vi "Main.vi"(8 "error in":errorcluster caption="entrée d'erreur") -> (0 "error out":errorcluster caption="sortie d'erreur")   [LabVIEW 2026]
uses:
  FGV_Controls/State.ctl
  FGV_Controls/TypeDef_FGV.ctl
panel:
  in  "Delete Positions":bool
  out "Multipositions":dbl[][](array[numeric])
  in  "Add":bool
  in  "Relative movement (mm)":dbl[](array[numeric]) format="%.6f"
  in  "Set Vel":bool
  in  "Velocity values":dbl[](array[numeric]) format="%.6f"
  out "Velocity":dbl[](array[numeric]) format="%.6f"
  in  "Mode":bool
  in  "Mov Rel":bool
  in  "Mov Abs":bool
  in  "Go to (mm)":dbl[](array[numeric]) format="%.6f"
  out "Current positions":dbl[](array[numeric])
  in  "Servo mode":bool[](array[boolean])
  out "+/- movement\nrange":dbl[](array[numeric]) format="%.6f"
  in  "Stop":bool
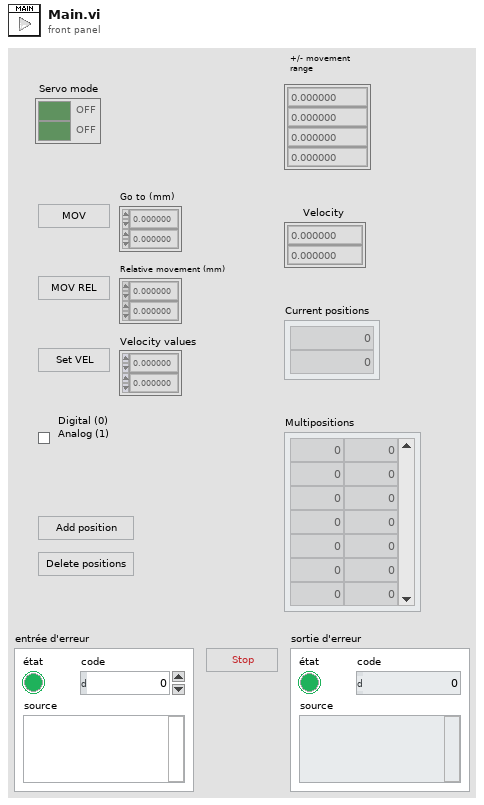
[diagram p1: front panel]
types:
  T1 = typedef "TypeDef_FGV.ctl" = enum16{"Initialize", "Write", "Read"}
  T2 = typedef "State.ctl" = enum16{"Initialize", "Wait for Event", "MOVAbs", "MOVRel", "SVO", "Analog-Digital", "POS?", "VEL", "STOP"}
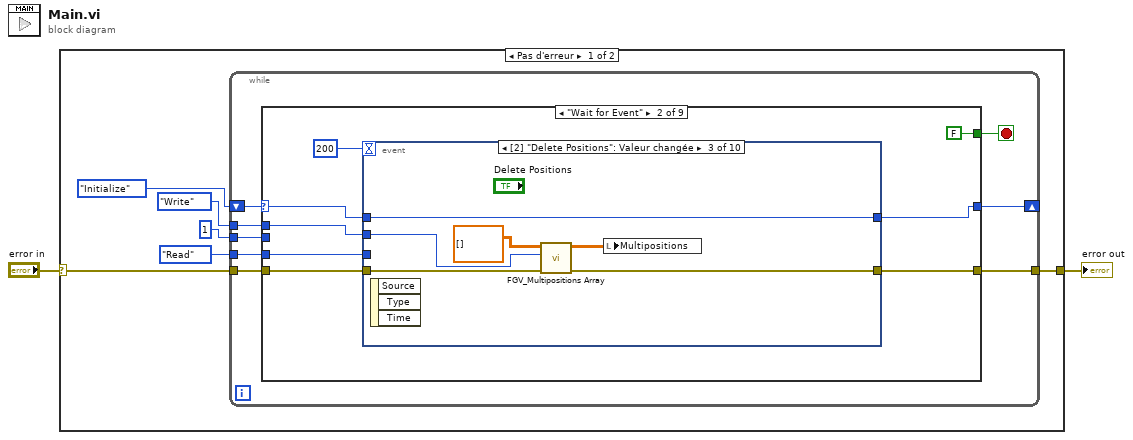
[diagram p0: block diagram]
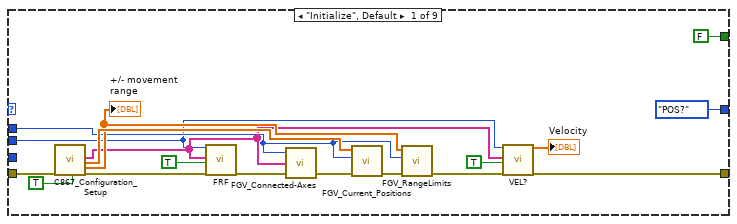
[diagram p2: hidden frame]
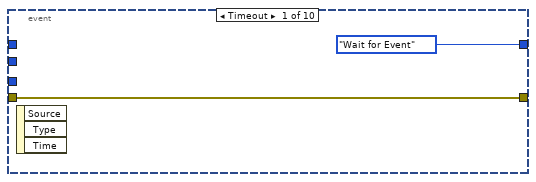
[diagram p3: hidden frame]
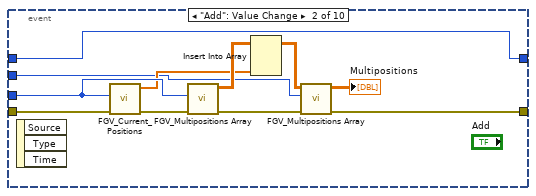
[diagram p4: hidden frame]
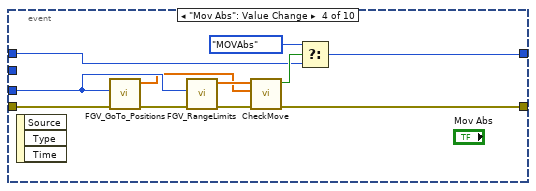
[diagram p5: hidden frame]
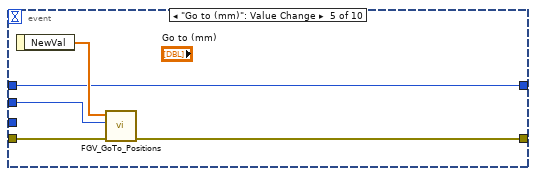
[diagram p6: hidden frame]
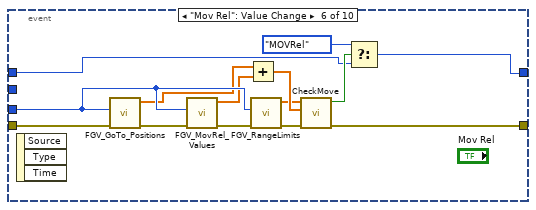
[diagram p7: hidden frame]
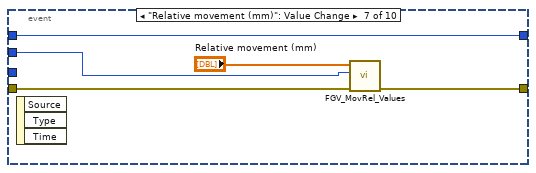
[diagram p8: hidden frame]
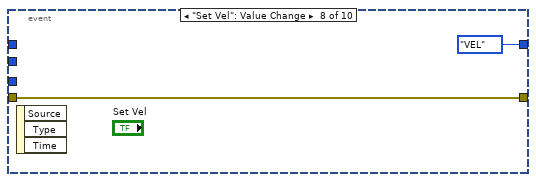
[diagram p9: hidden frame]
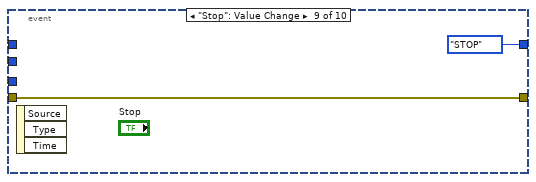
[diagram p10: hidden frame]
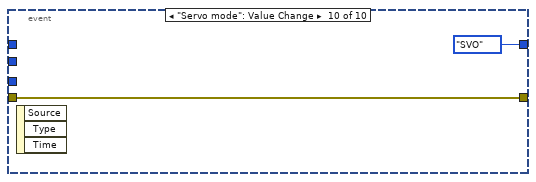
[diagram p11: hidden frame]
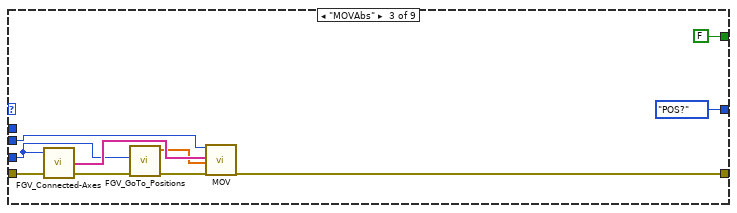
[diagram p12: hidden frame]
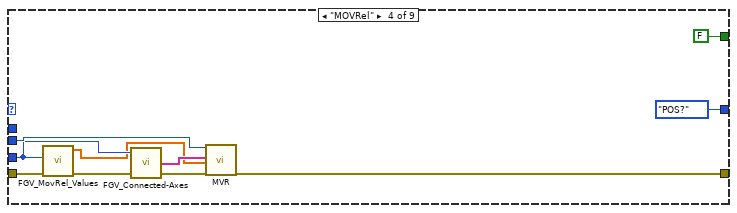
[diagram p13: hidden frame]
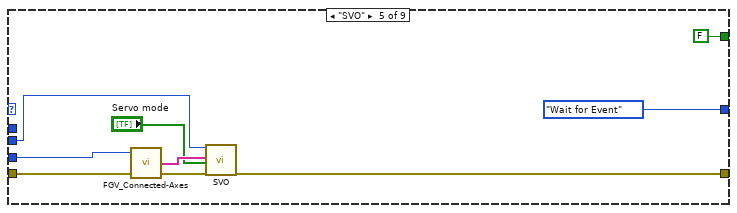
[diagram p14: hidden frame]
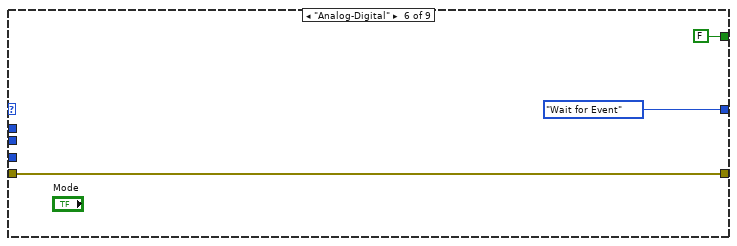
[diagram p15: hidden frame]
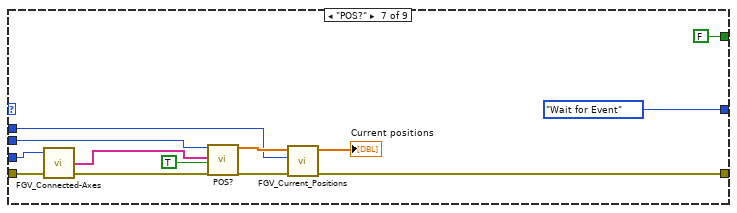
[diagram p16: hidden frame]
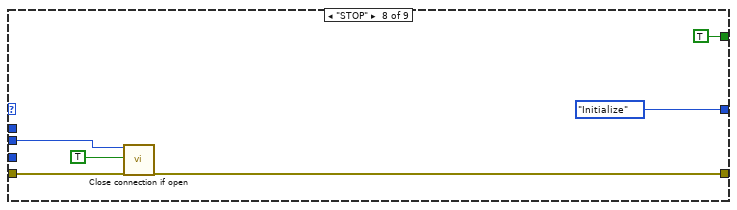
[diagram p17: hidden frame]
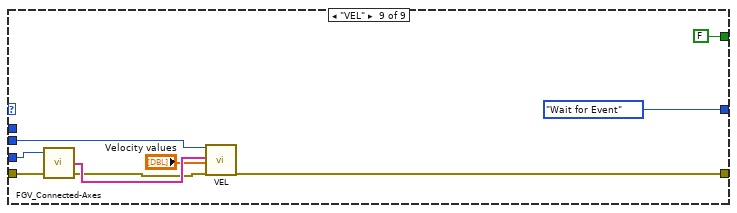
[diagram p18: hidden frame]
diagram:
  n1 = case shown="Pas d'erreur" "error in" {
    selector: "error in" -> [w7 w163]
    tunnel: [w6 w163] -> w1
    frame No Error {
      n2 = while {
        shift-right: [w15] -> _
        shift-left: State."Initialize" ("State") -> [w16]
        tunnel: w7 -> [w13]
        tunnel: [w12] -> w6
        tunnel: TypeDef_FGV."Write" ("Action") -> [w11]
        tunnel: TypeDef_FGV."Read" ("Action") -> [w10]
        tunnel: 1 ("System no.") -> [w9]
        stop <- w14 stop-if-true
        n3 = case shown="\"Wait for Event\"" w16 {
          selector: w16 -> [_ w42 _ _ _ _ _ _ _]
          tunnel: [State."POS?" ("State") w41 State."POS?" ("State") State."POS?" ("State") State."Wait for Event" ("State") State."Wait for Event" ("State") State."Wait for Event" ("State") State."Initialize" ("State") State."Wait for Event" ("State")] -> w15
          tunnel: [FALSE FALSE FALSE FALSE FALSE FALSE FALSE TRUE FALSE] -> w14
          tunnel: w13 -> [w32 w37 w110 w116 w129 w132 w145 w149 w159]
          tunnel: [w21 w38 w109 w120 w126 w132 w138 w148 w158] -> w12
          tunnel: w11 -> [w26 w36 _ _ _ _ w136 _ _]
          tunnel: w10 -> [_ w35 w104 w114 w124 _ w137 _ w162]
          tunnel: w9 -> [w17 _ w107 w117 w123 _ w135 w150 w154]
          frame "Initialize", Default {
            n4 = call "C867_Configuration_Setup.vi"("error in"=w32, "Switch servo on?"=TRUE) -> ("Conn. \nAxis"=w20:string[], "Position"=w29:dbl[], "+/- movement\nrange"=w27:dbl[], "error out"=w24:errorcluster)  [unwired: 11 in, 3 out]
            "+/- movement\nrange" <- w27
            n5 = call "FRF.vi"("System no."=w17, "Affected axes"=w20, "All axes?"=TRUE, "error in"=w24) -> ("error out"=w23:errorcluster)  [unwired: 15 in]
            n6 = call "FGV_Connected-Axes.vi"("error in"=w23, "Conn. \nAxis in"=w20, "Action"=w26) -> ("error out"=w30:errorcluster)  [unwired: 1 in, 1 out]
            n7 = call "FGV_Current_Positions.vi"("error in"=w30, "Action"=w26, "Current position IN"=w29) -> ("error out"=w28:errorcluster)  [unwired: 7 in, 1 out]
            n8 = call "FGV_RangeLimits.vi"("error in"=w28, "Action"=w26, "Range limits IN"=w27) -> ("error out"=w22:errorcluster)  [unwired: 7 in, 1 out]
            n9 = call "VEL?.vi"("System no."=w17, "Axes to query"=w20, "All axes?"=TRUE, "error in"=w22) -> ("Velocity"=→"Velocity":dbl[], "error out"=w21:errorcluster)  [unwired: 14 in]
          }
          frame "Wait for Event" {
            n10 = event shown="[2] \"Delete Positions\": Valeur changée" {
              selector: _ -> [_ _ _ _ _ _ _ _ _ _]
              dyn-events: _ -> [_ _ _ _ _ _ _ _ _ _]
              timeout: 200 -> [_ _ _ _ _ _ _ _ _ _]
              tunnel: w42 -> [_ w46 w58 w62 w73 w78 w92 _ _ _]
              tunnel: [State."Wait for Event" ("State") w46 w58 w63 w73 w80 w92 State."VEL" ("State") State."STOP" ("State") State."SVO" ("State")] -> w41
              tunnel: w37 -> [w43 w55 w61 w72 w77 w88 w94 w97 w99 w101]
              tunnel: [w43 w47 w60 w66 w76 w86 w93 w97 w99 w101] -> w38
              tunnel: w36 -> [_ w48 w56 _ w75 _ w95 _ _ _]
              tunnel: w35 -> [_ w53 _ w71 _ w87 _ _ _ _]
              event Timeout {
                n11 = event-data() -> ()  [unwired: 1 in, 3 out]
              }
              event "Add": Value Change {
                n12 = event-data() -> ()  [unwired: 1 in, 3 out]
                n13 = call "FGV_Current_Positions.vi"("error in"=w55, "Action"=w53) -> ("error out"=w54:errorcluster, "Current position array OUT"=w51:dbl[])  [unwired: 8 in]
                n14 = call "FGV_Multipositions Array.vi"("error in"=w54, "Action"=w53) -> ("error out"=w50:errorcluster, "Current position array OUT"=w52:dbl[][])  [unwired: 8 in]
                n15 = Insert Into Array(array=w52, new element=w51) -> (w49:dbl[][])  [unwired: 2 in]
                n16 = call "FGV_Multipositions Array.vi"("error in"=w50, "Action"=w48, "Current position IN"=w49) -> ("error out"=w47:errorcluster, "Current position array OUT"=→"Multipositions":dbl[][])  [unwired: 7 in]
              }
              event "Delete Positions": Value Change {
                n17 = event-data() -> ()  [unwired: 1 in, 3 out]
                n18 = call "FGV_Multipositions Array.vi"("error in"=w61, "Action"=w56, "Current position IN"=dbl[][] []) -> ("error out"=w60:errorcluster, "Current position array OUT"=w59:dbl[][])  [unwired: 7 in]
                n19 = local write "Multipositions"(w59) -> ()
              }
              event "Mov Abs": Value Change {
                n20 = event-data() -> ()  [unwired: 1 in, 3 out]
                n21 = call "FGV_GoTo_Positions.vi"("error in"=w72, "Action"=w71) -> ("error out"=w70:errorcluster, "GoTo position array OUT"=w67:dbl[])  [unwired: 8 in]
                n22 = call "FGV_RangeLimits.vi"("error in"=w70, "Action"=w71) -> ("error out"=w69:errorcluster, "Range limits array OUT"=w68:dbl[])  [unwired: 8 in]
                n23 = call "CheckMove.vi"("error in"=w69, "Go to (mm)"=w67, "Limits"=w68) -> ("error out"=w66:errorcluster, "Validated!"=w65:bool)  [unwired: 7 in]
                n24 = Select(t=State."MOVAbs" ("State"), s=w65, f=w62) -> (s? t:f=w63:T2)
              }
              event "Go to (mm)": Value Change {
                n25 = event-data() -> ("NewVal"=w74:dbl[])  [unwired: 1 in]
                n26 = call "FGV_GoTo_Positions.vi"("error in"=w77, "Action"=w75, "GoTo position IN"=w74) -> ("error out"=w76:errorcluster)  [unwired: 7 in, 1 out]
              }
              event "Mov Rel": Value Change {
                n27 = event-data() -> ()  [unwired: 1 in, 3 out]
                n28 = call "FGV_GoTo_Positions.vi"("error in"=w88, "Action"=w87) -> ("error out"=w91:errorcluster, "GoTo position array OUT"=w85:dbl[])  [unwired: 8 in]
                n29 = call "FGV_MovRel_Values.vi"("error in"=w91, "Action"=w87) -> ("error out"=w90:errorcluster, "MovRel position array OUT"=w84:dbl[])  [unwired: 8 in]
                n30 = Add(x=w85, y=w84) -> (x+y=w83:dbl[])
                n31 = call "FGV_RangeLimits.vi"("error in"=w90, "Action"=w87) -> ("error out"=w89:errorcluster, "Range limits array OUT"=w82:dbl[])  [unwired: 8 in]
                n32 = call "CheckMove.vi"("error in"=w89, "Go to (mm)"=w83, "Limits"=w82) -> ("error out"=w86:errorcluster, "Validated!"=w79:bool)  [unwired: 7 in]
                n33 = Select(t=State."MOVRel" ("State"), s=w79, f=w78) -> (s? t:f=w80:T2)
              }
              event "Relative movement (mm)": Value Change {
                n34 = event-data() -> ()  [unwired: 1 in, 3 out]
                n35 = call "FGV_MovRel_Values.vi"("error in"=w94, "Action"=w95, "MovRel position IN"="Relative movement (mm)") -> ("error out"=w93:errorcluster)  [unwired: 7 in, 1 out]
              }
              event "Set Vel": Value Change {
                n36 = event-data() -> ()  [unwired: 1 in, 3 out]
              }
              event "Stop": Value Change {
                n37 = event-data() -> ()  [unwired: 1 in, 3 out]
              }
              event "Servo mode": Value Change {
                n38 = event-data() -> ()  [unwired: 1 in, 3 out]
              }
            }
          }
          frame "MOVAbs" {
            n39 = call "FGV_Connected-Axes.vi"("error in"=w110, "Action"=w104) -> ("error out"=w106:errorcluster, "Conn. \nAxis out"=w108:string[])  [unwired: 2 in]
            n40 = call "FGV_GoTo_Positions.vi"("error in"=w106, "Action"=w104) -> ("error out"=w105:errorcluster, "GoTo position array OUT"=w103:dbl[])  [unwired: 8 in]
            n41 = call "MOV.vi"("System no."=w107, "Axes to move"=w108, "Position values"=w103, "error in"=w105) -> ("error out"=w109:errorcluster)  [unwired: 15 in]
          }
          frame "MOVRel" {
            n42 = call "FGV_MovRel_Values.vi"("error in"=w116, "Action"=w114) -> ("error out"=w115:errorcluster, "MovRel position array OUT"=w113:dbl[])  [unwired: 8 in]
            n43 = call "FGV_Connected-Axes.vi"("error in"=w115, "Action"=w114) -> ("error out"=w118:errorcluster, "Conn. \nAxis out"=w119:string[])  [unwired: 2 in]
            n44 = call "MVR.vi"("System no."=w117, "Axes to move"=w119, "Position values"=w113, "error in"=w118) -> ("error out"=w120:errorcluster)  [unwired: 15 in]
          }
          frame "SVO" {
            n45 = call "FGV_Connected-Axes.vi"("error in"=w129, "Action"=w124) -> ("error out"=w127:errorcluster, "Conn. \nAxis out"=w128:string[])  [unwired: 2 in]
            n46 = call "SVO.vi"("System no."=w123, "Axes to command"=w128, "Servo mode"="Servo mode", "error in"=w127) -> ("error out"=w126:errorcluster)  [unwired: 15 in]
          }
          frame "Analog-Digital" {
          }
          frame "POS?" {
            n47 = call "FGV_Connected-Axes.vi"("error in"=w145, "Action"=w137) -> ("error out"=w142:errorcluster, "Conn. \nAxis out"=w144:string[])  [unwired: 2 in]
            n48 = call "POS?.vi"("System no."=w135, "Axes to query"=w144, "All axes?"=TRUE, "error in"=w142) -> ("Position"=w140:dbl[], "error out"=w141:errorcluster)  [unwired: 14 in]
            n49 = call "FGV_Current_Positions.vi"("error in"=w141, "Action"=w136, "Current position IN"=w140) -> ("error out"=w138:errorcluster, "Current position array OUT"=→"Current positions":dbl[])  [unwired: 7 in]
          }
          frame "STOP" {
            n50 = call "Close connection if open.vi"("System no."=w150, "Close DaisyChain"=TRUE, "error in"=w149) -> ("error out"=w148:errorcluster)  [unwired: 15 in, 1 out]
          }
          frame "VEL" {
            n51 = call "FGV_Connected-Axes.vi"("error in"=w159, "Action"=w162) -> ("error out"=w160:errorcluster, "Conn. \nAxis out"=w161:string[])  [unwired: 2 in]
            n52 = call "VEL.vi"("System no."=w154, "Axes to set"=w161, "Velocity values"="Velocity values", "error in"=w160) -> ("error out"=w158:errorcluster)  [unwired: 14 in, 1 out]
          }
        }
      }
    }
    frame Error {
    }
  }
  "error out" <- w1
